vi "test Connector Pane.vi"(8 "error in (no error)":errorcluster, 11 "TestCase in":refnum<class "Ballard ARINC 429 Unit Tests.lvclass">) -> (0 "error out":errorcluster, 3 "TestCase out":refnum<class "Ballard ARINC 429 Unit Tests.lvclass">)   [LabVIEW 2020, in "Ballard ARINC 429 Unit Tests.lvclass"]
uses:
  Ballard ARINC 429 Unit Tests.lvclass
  <vilib>/addons/_JKI Toolkits/VI Tester/TestCase.llb/TestCase.lvclass
  niveristand-custom-device-testing-tools/VeriStandTestUtilities/VeriStandTestUtilities.lvlib
  C:/Program Files (x86)/National Instruments/LabVIEW 2020/vi.lib/addons/_JKI Toolkits/VI Tester/TestCase.llb/TestCase.lvclass
  C:/Users/nitest/Desktop/Git 2020/niveristand-ballard-arinc429-custom-device/Source/Custom Device/Tests/Unit/Ballard ARINC 429 Unit Tests.lvclass
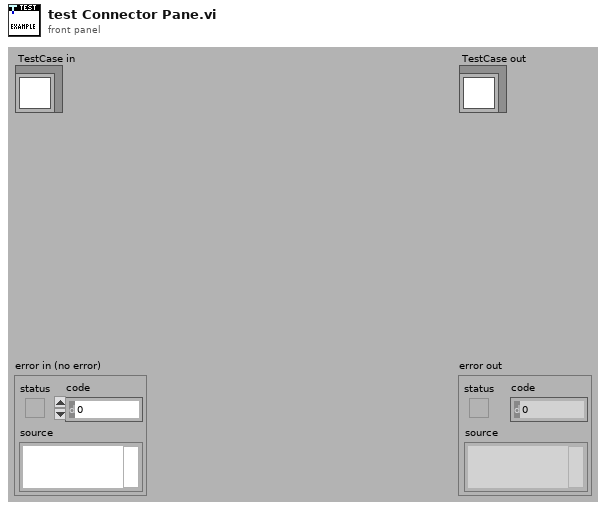
[diagram p1: front panel]
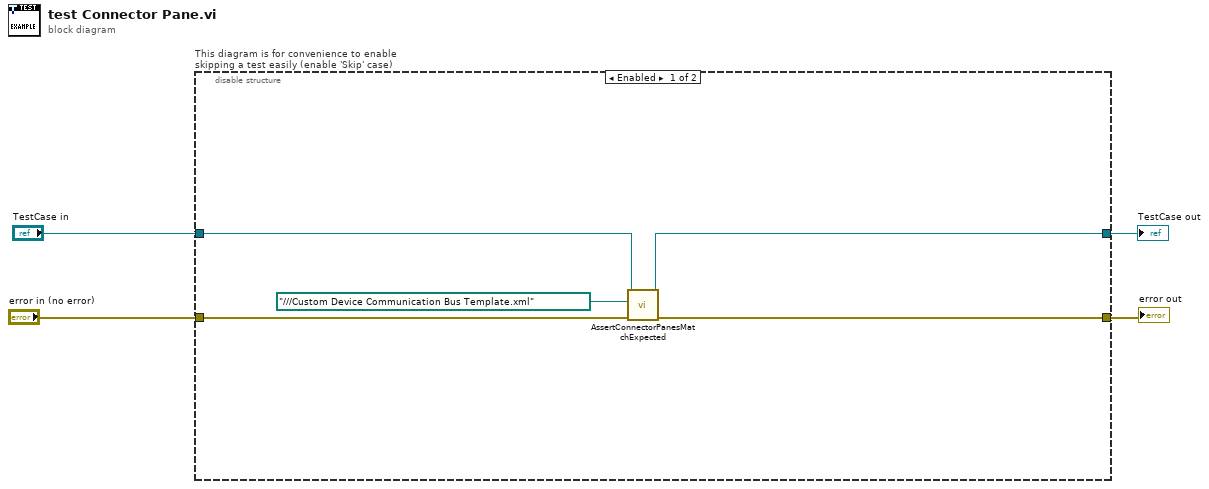
[diagram p0: block diagram]
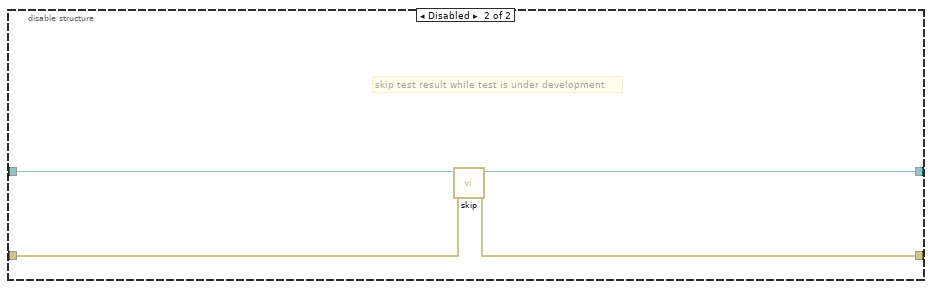
[diagram p2: hidden frame]
diagram:
  n1 = disable-structure "This diagram is for convenience to enable skipping a test easily (enable 'Skip' case)" shown="Enabled" {
    disable-tunnel: "TestCase in" -> [w7 w13]
    disable-tunnel: [w6 w11] -> w1
    disable-tunnel: [w8 w12] -> w3
    disable-tunnel: "error in (no error)" -> [w9 w10]
    frame Enabled {
      n2 = call "AssertConnectorPanesMatchExpected.vi"("error in (no error)"=w9, "custom device xml path"=path "../../../Custom Device Communication Bus Template.xml", "TestCase in"=w7) -> ("error out"=w8:errorcluster, "TestCase out"=w6:refnum<class "Ballard ARINC 429 Unit Tests.lvclass">)  [unwired: 7 in]
    }
    frame Disabled {
      # "skip test result while test is under development"
      n3 = call <vilib>:"skip.vi"("error in (no error)"=w10, "TestCase in"=w13) -> ("error out"=w12:errorcluster, "TestCase out"=w11:refnum<class "Ballard ARINC 429 Unit Tests.lvclass">)  [unwired: 8 in]
    }
  }
  "error out" <- w3
  "TestCase out" <- w1
